vi "Run CC.vi"(8 "error in (no error)":errorcluster, 10 "Run":T1, 11 "Camera Controller in":refnum<class "Camera Controller.lvclass">) -> (0 "error out":errorcluster, 3 "Camera Controller out":refnum<class "Camera Controller.lvclass">)   [LabVIEW 2019, in "Camera Controller.lvlib" / "Camera Controller.lvclass"]
uses:
  Camera Controller.lvclass
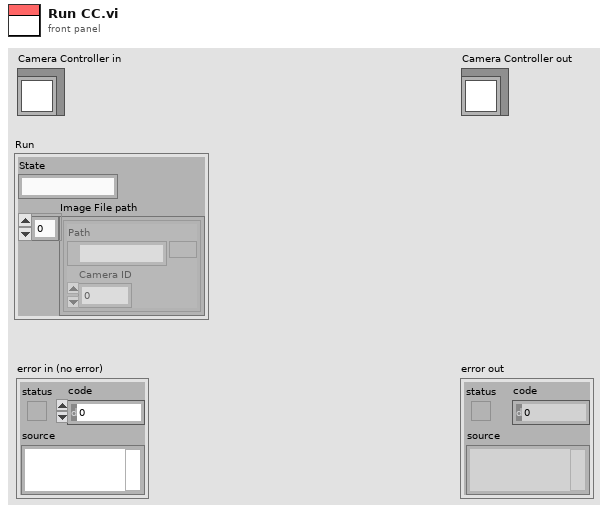
[diagram p1: front panel]
types:
  T1 = cluster{"State":string, "Image File path":cluster{"Path":path, "Camera ID":i32}[]}
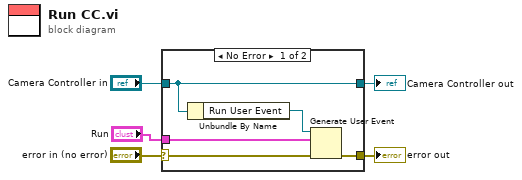
[diagram p0: block diagram]
diagram:
  n1 = case shown="No Error" "error in (no error)" {
    selector: "error in (no error)" -> [w9 w12]
    tunnel: [w8 w12] -> w4
    tunnel: [w10 w11] -> w2
    tunnel: "Camera Controller in" -> [w10 w11]
    tunnel: "Run" -> [w7 _]
    frame No Error {
      n2 = Unbundle By Name(w10) -> ("Run User Event"=w6:refnum<user-event>)
      n3 = Generate User Event(user event=w6, event data cluster=w7, error in=w9) -> (error out=w8:errorcluster)  [unwired: 1 in, 1 out]
    }
    frame Error {
    }
  }
  "error out" <- w4
  "Camera Controller out" <- w2
